vi "Configure Offset.vi"(5 "Offset Value (0 dB)":dbl, 7 "Enable Offset (F: Disable)":bool, 8 "error in (no error)":errorcluster, 11 "VISA resource name":refnum<visa-resource-name>) -> (0 "error out":errorcluster, 3 "VISA resource name out":refnum<visa-resource-name>)   [LabVIEW 2014, in "Agilent U2000 Series.lvlib"]
doc: "Configures the offset which is used to compensate for gain and loss."
uses:
  Agilent U2000 Series.lvlib
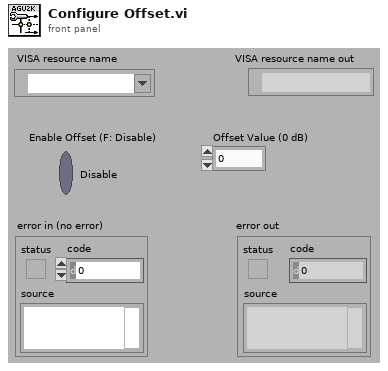
[diagram p1: front panel]
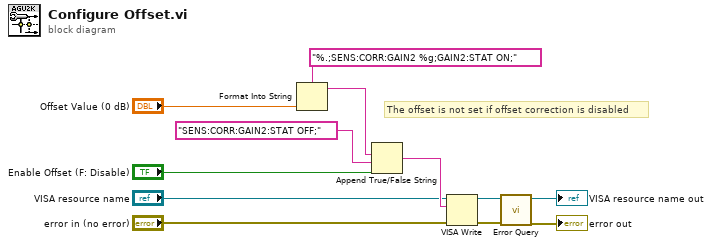
[diagram p0: block diagram]
diagram:
  # "The offset is not set if offset correction is disabled"
  n1 = Format Into String(format string="%.;SENS:CORR:GAIN2 %g;GAIN2:STAT ON;", "Offset Value (0 dB)") -> (resulting string=w5:string)  [unwired: 2 in, 1 out]
  n2 = Append True/False String(1:"Enable Offset (F: Disable)", 2:"SENS:CORR:GAIN2:STAT OFF;", 3:w5) -> (0:w9:string)  [unwired: 1 out]
  n3 = VISA Write(VISA resource name="VISA resource name", write buffer=w9, error in (no error)="error in (no error)") -> (VISA resource name out=w3:refnum<visa-resource-name>, error out=w4:errorcluster)  [unwired: 1 out]
  n4 = call "Error Query.vi"("error in (no error)"=w4, "VISA resource name"=w3) -> ("error out"=→"error out":errorcluster, "VISA resource name out"=→"VISA resource name out":refnum<visa-resource-name>)  [unwired: 8 out]
